vi "PicoScope5000aPowerSource.vi"(6 "USB 3.0 on non-USB 3.0 port control":bool=TRUE, 7 "Mode":u16(ring) items=["Dialog On Error", "no dialog - CloseUnit and Stop", "no dialog - Continue", "no dialog - Stop"], 8 "USB Powered control":bool=TRUE, 9 "handle in":i16, 10 "PICO STATUS IN":u32 format="%#.0f", 11 "error in (no error)":errorcluster) -> (0 "USB Powered":bool=TRUE, 1 "handle out":i16, 2 "PICO STATUS OUT":u32, 3 "error out":errorcluster, 4 "USB 3.0 on non-USB 3.0 Port":bool=TRUE)   [LabVIEW 2017]
uses:
  ps5000a.dll
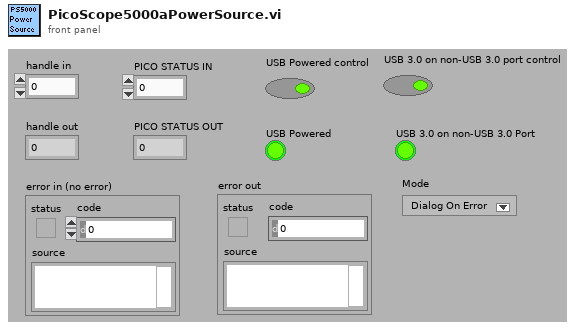
[diagram p1: front panel]
types:
  T1 = cluster{"status":bool, "code":u32, "source":string}
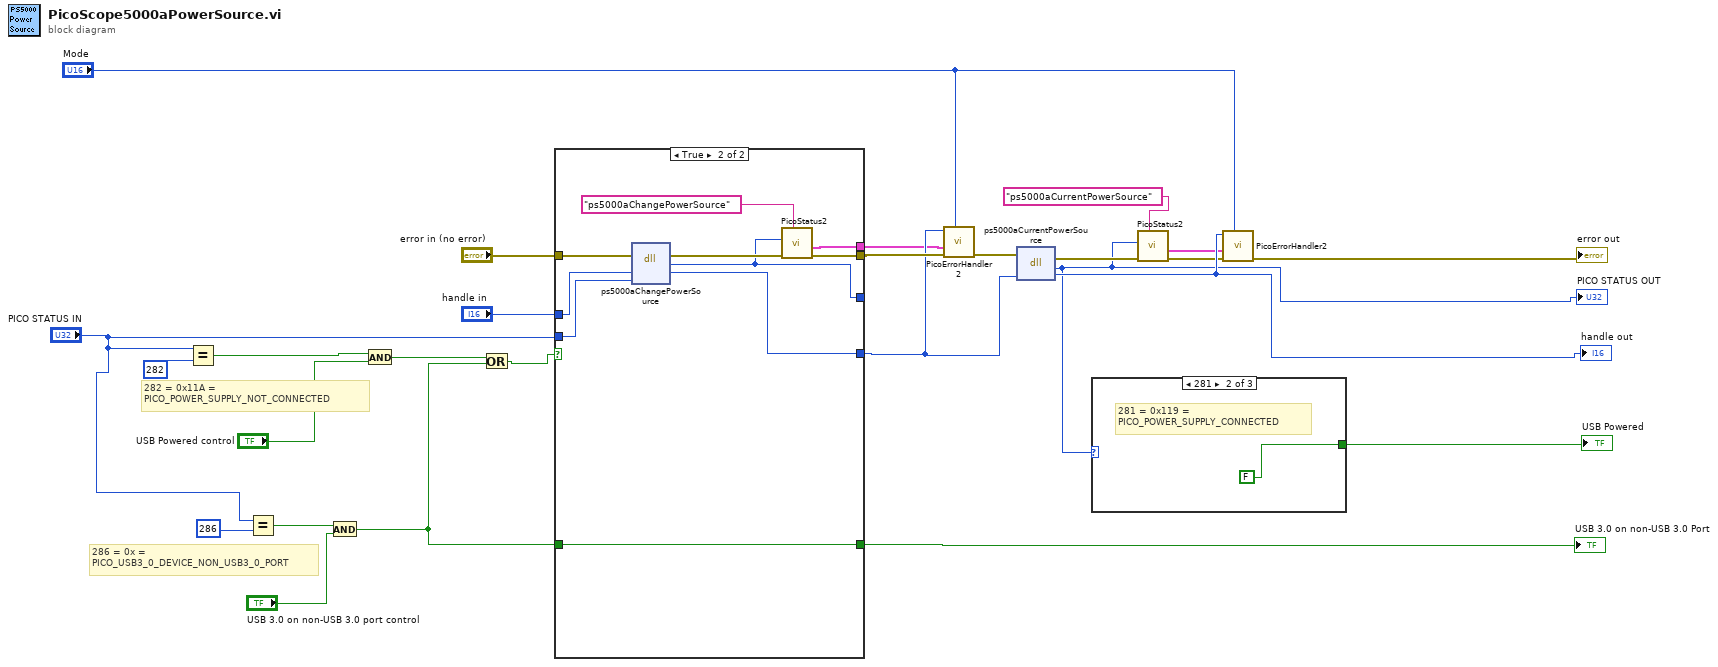
[diagram p0: block diagram]
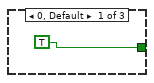
[diagram p2: hidden frame]
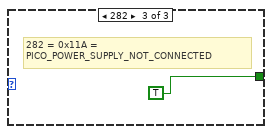
[diagram p3: hidden frame]
diagram:
  # "286 = 0x = \nPICO_USB3_0_DEVICE_NON_USB3_0_PORT"
  # "282 = 0x11A = \nPICO_POWER_SUPPLY_NOT_CONNECTED"
  n1 = Equal?(x="PICO STATUS IN", y=u32 282) -> (x = y?=w25:bool)
  n2 = Equal?(x="PICO STATUS IN", y=u32 286) -> (x = y?=w21:bool)
  n3 = And(x=w21, y="USB 3.0 on non-USB 3.0 port control") -> (x .and. y?=w8:bool)
  n4 = And(x=w25, y="USB Powered control") -> (x .and. y?=w18:bool)
  n5 = Or(x=w18, y=w8) -> (x .or. y?=w17:bool)
  n6 = case shown="True" w17 {
    tunnel: "PICO STATUS IN" -> [w30 w39]
    tunnel: [w30 w33] -> _
    tunnel: [w29 w35] -> w12
    tunnel: "error in (no error)" -> [w29 w40]
    tunnel: "handle in" -> [w28 w38]
    tunnel: [w28 w37] -> w11
    tunnel: w8 -> [w27 w36]
    tunnel: [w27 w36] -> w15
    tunnel: [_ w31] -> w2
    frame False {
    }
    frame True {
      n7 = dll-call lib="ps5000a.dll" fn="ps5000aChangePowerSource"(error in=w40, "handle"=w38, "powerSource"=w39) -> (error out=w34:errorcluster, "PICO_STATUS"=w33:u32, "handle"=w37:i16)  [unwired: 3 in, 1 out]
      n8 = call "PicoStatus2.vi"("PICO source"="ps5000aChangePowerSource" ("source"), "Error in"=w34, "PICO STATUS"=w33) -> ("error out"=w35:errorcluster, "PICO_STATUS out"=w31:T1)  [unwired: 5 in]
    }
  }
  "USB 3.0 on non-USB 3.0 Port" <- w15
  n9 = call "PicoErrorHandler2.vi"("Mode"="Mode", "error in (no error)"=w12, "PICO_STATUS in"=w2, "handle In"=w11) -> ("error out"=w14:errorcluster)  [unwired: 7 in]
  n10 = dll-call lib="ps5000a.dll" fn="ps5000aCurrentPowerSource"(error in=w14, "handle"=w11) -> (error out=w6:errorcluster, "PICO_STATUS"=w3:u32, "handle"=w10:i16)  [unwired: 2 in, 1 out]
  "PICO STATUS OUT" <- w3
  "handle out" <- w10
  n11 = case shown="281" w3 {
    tunnel: [TRUE FALSE TRUE] -> w9
    frame 0, Default {
    }
    frame 281 {
      # "281 = 0x119 = \nPICO_POWER_SUPPLY_CONNECTED"
    }
    frame 282 {
      # "282 = 0x11A = \nPICO_POWER_SUPPLY_NOT_CONNECTED"
    }
  }
  "USB Powered" <- w9
  n12 = call "PicoStatus2.vi"("PICO source"="ps5000aCurrentPowerSource" ("source"), "Error in"=w6, "PICO STATUS"=w3) -> ("error out"=w7:errorcluster, "PICO_STATUS out"=w4:T1)  [unwired: 5 in]
  n13 = call "PicoErrorHandler2.vi"("Mode"="Mode", "error in (no error)"=w7, "PICO_STATUS in"=w4, "handle In"=w10) -> ("error out"=→"error out":errorcluster)  [unwired: 7 in]
